vi "bool_to_enable_state.vi"(5 "boolean in":bool=TRUE) -> (2 "enabled status out":T1(ring))   [LabVIEW 2010]
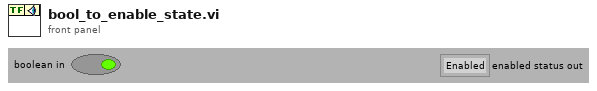
[diagram p1: front panel]
types:
  T1 = enum8{"Enabled", "Disabled", "Disabled and Grayed Out"}
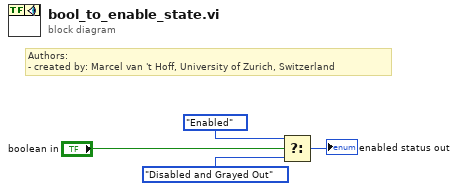
[diagram p0: block diagram]
diagram:
  # "Authors: \n- created by: Marcel van 't Hoff, University of Zurich, Switzerland"
  n1 = Select(t=T1."Enabled" ("Disabled"), s="boolean in", f=T1."Disabled and Grayed Out" ("Disabled")) -> (s? t:f=→"enabled status out":T1)
